vi "mod_Weighted Linear Fit.vi"(7 "reset?":bool, 8 "weights":dbl[](array[numeric]) format="%.2f", 10 "X Values":dbl[](array[numeric]) format="%.2f", 11 "Y Values":dbl[](array[numeric]) format="%.2f") -> (0 "intercept":dbl format="%.2f", 1 "slope":dbl format="%.2f", 3 "weighted linear fit":dbl[](array[numeric]) format="%.2f")   [LabVIEW 2020, in "niAMT.lvlib"]
uses:
  <vilib>/addons/Modulation/niAMT.lvlib
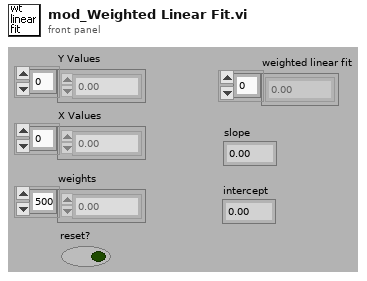
[diagram p1: front panel]
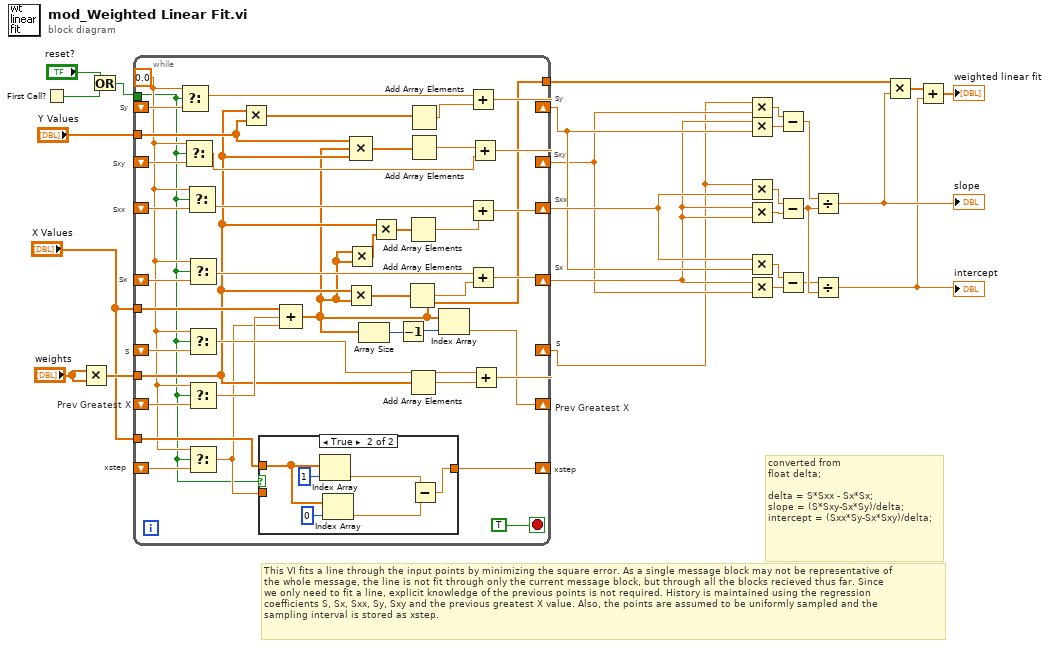
[diagram p0: block diagram]
diagram:
  # "converted from \nfloat delta;\n\ndelta = S*Sxx - Sx*Sx;\nslope = (S*Sxy-Sx*Sy)/delta;\nintercept = (Sxx*Sy-Sx*Sxy)/delta;"
  # "This VI fits a line through the input points by minimizing the square error. As a single message block may not be representative of\nthe whole message, the line is not fit through only the current message block, but through all the blocks recieved thus far. Since\nwe only need to fit a line, explicit knowledge of the previous points is not required. History is maintained using the regression \ncoefficients S, Sx, Sxx, Sy, Sxy and the previous greatest X value. Also, the points are assumed to be uniformly sampled and the\nsampling interval is stored as xstep."
  # "xstep"
  # "S"
  # "Prev Greatest X"
  # "Sx"
  # "Sxx"
  # "Sxy"
  # "Sy"
  # "xstep"
  # "S"
  # "Prev Greatest X"
  # "Sx"
  # "Sxx"
  # "Sxy"
  # "Sy"
  n1 = First Call?() -> (First Call?: T/F=w18:bool)
  n2 = Multiply(x="weights", y="weights") -> (x*y=w25:dbl[])
  n3 = Or(x="reset?", y=w18) -> (x .or. y?=w17:bool)
  n4 = while {
    shift-right: [w32] -> w4
    shift-left: _ -> [w54]
    shift-right: [w39] -> w2
    shift-left: _ -> [w55]
    shift-right: [w42] -> w5
    shift-left: _ -> [w56]
    shift-right: [w47] -> w3
    shift-left: _ -> [w57]
    shift-right: [w51] -> _
    shift-left: _ -> [w60]
    shift-right: [w61] -> w1
    shift-left: _ -> [w64]
    shift-right: [w66] -> _
    shift-left: _ -> [w29]
    tunnel: "X Values" -> [w65]
    tunnel: w25 -> [w37]
    tunnel: "X Values" -> [w58]
    tunnel: "Y Values" -> [w38]
    tunnel: [w31] -> w21
    tunnel: w17 -> [w27]
    stop <- TRUE stop-if-true
    w30 = 0.0
    n5 = Select(t=w30, s=w27, f=w54) -> (s? t:f=w33:dbl)
    n6 = Select(t=w30, s=w27, f=w55) -> (s? t:f=w41:dbl)
    n7 = Select(t=w30, s=w27, f=w56) -> (s? t:f=w43:dbl)
    n8 = Select(t=w30, s=w27, f=w57) -> (s? t:f=w48:dbl)
    n9 = Select(t=w30, s=w27, f=w64) -> (s? t:f=w63:dbl)
    n10 = Select(t=w30, s=w27, f=w60) -> (s? t:f=w59:dbl)
    n11 = Select(t=w30, s=w27, f=w29) -> (s? t:f=w28:dbl)
    n12 = Multiply(x=w37, y=w38) -> (x*y=w35:dbl[])
    n13 = case shown="True" w27 {
      tunnel: w28 -> [w68 _]
      tunnel: [w68 w69] -> w66
      tunnel: w65 -> [_ w74]
      frame False {
      }
      frame True {
        n14 = Index Array(array=w74, index=1) -> (element=w71:dbl)
        n15 = Index Array(array=w74, index=0) -> (element=w70:dbl)
        n16 = Subtract(x=w71, y=w70) -> (x-y=w69:dbl)
      }
    }
    n17 = Compound Arithmetic op=unknown(w58, w59, w28) -> (w31:dbl[])
    n18 = Multiply(x=w37, y=w31) -> (x*y=w50:dbl[])
    n19 = Multiply(x=w31, y=w31) -> (x*y=w46:dbl[])
    n20 = Compound Arithmetic op=MULTIPLY(w38, w31, w37) -> (w36:dbl[])
    n21 = Array Size(array=w31) -> (size(s)=w53:i32)
    n22 = Multiply(x=w37, y=w46) -> (x*y=w45:dbl[])
    n23 = Decrement(x=w53) -> (x-1=w52:i32)
    n24 = Add Array Elements(numeric array=w50) -> (sum=w49:dbl)
    n25 = Add Array Elements(numeric array=w45) -> (sum=w44:dbl)
    n26 = Add Array Elements(numeric array=w37) -> (sum=w62:dbl)
    n27 = Add Array Elements(numeric array=w35) -> (sum=w34:dbl)
    n28 = Add Array Elements(numeric array=w36) -> (sum=w40:dbl)
    n29 = Index Array(array=w31, index=w52) -> (element=w51:dbl)
    n30 = Add(x=w33, y=w34) -> (x+y=w32:dbl)
    n31 = Add(x=w43, y=w44) -> (x+y=w42:dbl)
    n32 = Add(x=w48, y=w49) -> (x+y=w47:dbl)
    n33 = Add(x=w40, y=w41) -> (x+y=w39:dbl)
    n34 = Add(x=w63, y=w62) -> (x+y=w61:dbl)
  }
  n35 = Multiply(x=w1, y=w2) -> (x*y=w14:dbl)
  n36 = Multiply(x=w3, y=w4) -> (x*y=w15:dbl)
  n37 = Multiply(x=w1, y=w5) -> (x*y=w16:dbl)
  n38 = Multiply(x=w3, y=w3) -> (x*y=w13:dbl)
  n39 = Multiply(x=w5, y=w4) -> (x*y=w10:dbl)
  n40 = Multiply(x=w3, y=w2) -> (x*y=w9:dbl)
  n41 = Subtract(x=w14, y=w15) -> (x-y=w12:dbl)
  n42 = Subtract(x=w16, y=w13) -> (x-y=w11:dbl)
  n43 = Subtract(x=w10, y=w9) -> (x-y=w8:dbl)
  n44 = Divide(x=w12, y=w11) -> (x/y=w7:dbl)
  "slope" <- w7
  n45 = Divide(x=w8, y=w11) -> (x/y=w6:dbl)
  "intercept" <- w6
  n46 = Multiply(x=w21, y=w7) -> (x*y=w22:dbl[])
  n47 = Add(x=w22, y=w6) -> (x+y=→"weighted linear fit":dbl[])
